vi "Channel_Get_WfmPath.vi"(8 "error in (no error)":errorcluster, 11 "Channel in":refnum<class "Channel.lvclass">) -> (0 "error out":errorcluster, 2 "WfmPath":string, 3 "Channel out":refnum<class "Channel.lvclass">)   [LabVIEW 2023, in "Channel.lvclass"]
doc: "Get the path of the waveform source for this channel."
uses:
  Channel.lvclass
  Channel.lvclass/Channel.ctl
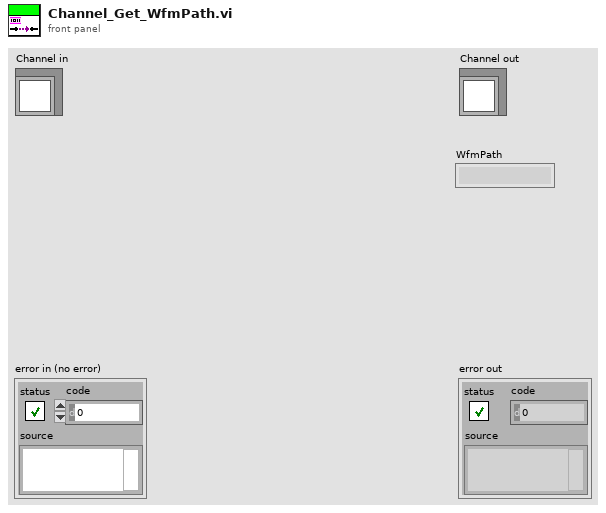
[diagram p1: front panel]
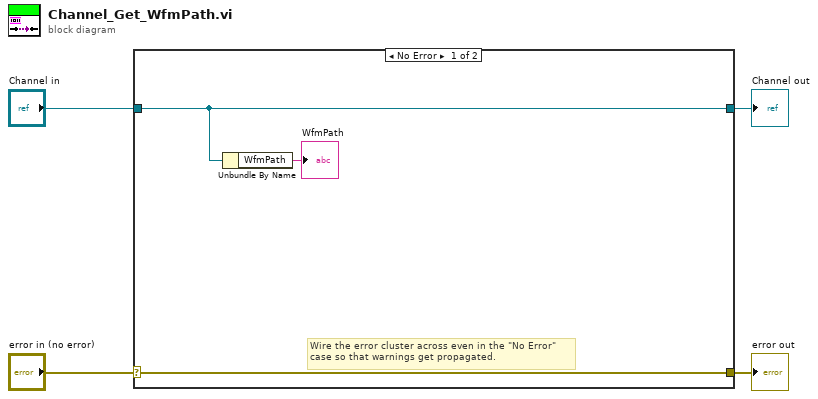
[diagram p0: block diagram]
diagram:
  n1 = case shown="No Error" "error in (no error)" {
    selector: "error in (no error)" -> [w7 w9]
    tunnel: [w7 w9] -> w3
    tunnel: [w6 w8] -> w1
    tunnel: "Channel in" -> [w6 w8]
    frame No Error {
      # "Wire the error cluster across even in the \"No Error\"\ncase so that warnings get propagated."
      n2 = Unbundle By Name(w6) -> ("WfmPath"=→"WfmPath":string)
    }
    frame Error {
    }
  }
  "error out" <- w3
  "Channel out" <- w1
